vi "PID Online Autotuning.vi"   [LabVIEW 2020, in "NI_PID_autopid.lvlib"]
doc: "Controls the parameters of a PID controller based on the autotuning technique of the polymorphic instance you select. You can use this VI in applications with other PID VIs, such as PID or PID Advanced, to construct and tune a PID controller. You must manually select the polymorphic instance to use."
uses:
  <vilib>/addons/control/pid/NI_PID_autopid.lvlib
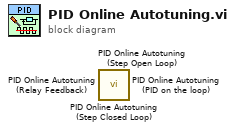
[diagram p0: block diagram]
diagram:
  n1 = call <vilib>:"PID Online Autotuning (Step Closed Loop).VI"() -> ()  [unwired: 11 in, 5 out]
  n2 = call <vilib>:"PID Online Autotuning (Step Open Loop).VI"() -> ()  [unwired: 11 in, 5 out]
  n3 = call <vilib>:"PID Online Autotuning (Relay Feedback).VI"() -> ()  [unwired: 11 in, 5 out]
  n4 = call <vilib>:"PID Online Autotuning (PID on the loop).VI"() -> ()  [unwired: 11 in, 5 out]
